vi "ConvertWaveGraphDataToListCtrl.vi"(11 "display graph":refnum<vi>) -> (3 "data":string[][](array[string]))   [LabVIEW 2018]
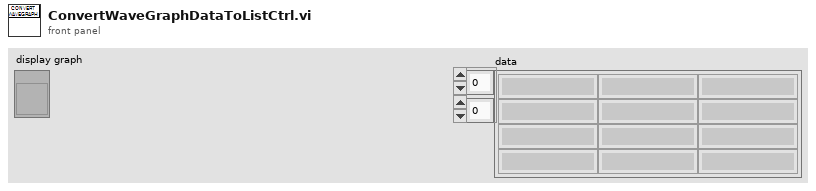
[diagram p1: front panel]
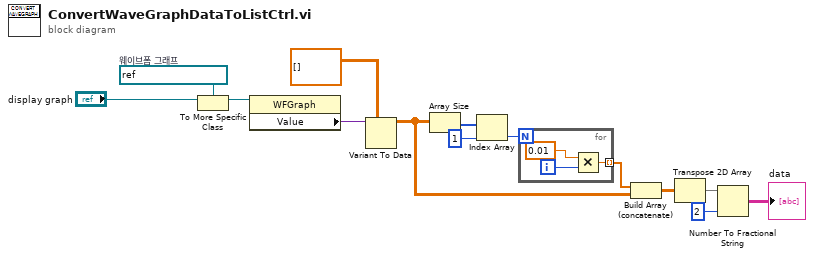
[diagram p0: block diagram]
diagram:
  w13 = refnum<vi> refnum  # 웨이브폼 그래프
  n1 = To More Specific Class(target class=w13, reference="display graph") -> (specific class reference=w12:refnum<vi>)  [unwired: 1 in, 1 out]
  n2 = property class="WFGraph"(reference=w12) -> ("Value"=w11:variant)  [unwired: 1 in, 2 out]
  n3 = Variant To Data(type=dbl[][] [] ("display Graph"), Variant=w11) -> (data=w4:dbl[][])  [unwired: 1 in, 1 out]
  n4 = Array Size(array=w4) -> (size(s)=w6:i32[])
  n5 = Index Array(array=w6, index=1 ("인덱스")) -> (element=w3:i32)
  n6 = for {
    N: w3 -> [_]
    tunnel: [w15] -> w2 mode=indexing
    i -> [w16]
    n7 = Multiply(x=0.01, y=w16) -> (x*y=w15:dbl)
  }
  n8 = Build Array (concatenate)(w2, w4) -> (w9:dbl[][])
  n9 = Transpose 2D Array(2D array=w9) -> (transposed array=w8:dbl[][])
  n10 = Number To Fractional String(number=w8, precision (6)=i16 2 ("정밀도(6)")) -> (F-format string=→"data":string[][])  [unwired: 2 in]
